vi "Configure Channel (OHM Scale).vi"(0 "VISA resource name":refnum<visa-resource-name>, 1 "Scaling":T2={"Floating point position (2)"=2, "Lower Scaling (0)"=0.0, "Upper Scaling (100.00)"=100.0, "Unit Character (\"\")"=""} {"Upper Scaling (100.00)" format="%_6g"; "Lower Scaling (0)" format="%_6g"; "Floating point position (2)" min=0 max=5 step=1}, 5 "Channel (0001)":string="0001", 7 "Enable Channel (True)":bool=TRUE, 9 "Type and Span":T1={"OHM Type (0 : 20ohm)"=0, "Enable Span (False)"=FALSE, "Lower Span (0.000)"=0.0, "Upper Span (20.000)"=20.0, "Bias (0)"=0.0} {"Bias (0)" format="%_6g"; "Upper Span (20.000)" min=-99999.0 max=99999.0 step=0.1 format="%.2f"; "Lower Span (0.000)" min=-99999.0 max=99999.0 step=0.1 format="%.2f"; "OHM Type (0 : 20ohm)" items=["20ohm", "200ohm", "2000ohm"]}, 11 "error in (no error)":errorcluster) -> (4 "VISA resource name out":refnum<visa-resource-name>, 6 "channel":string, 15 "error out":errorcluster)   [LabVIEW 2020, in "Yokogawa GX Series.lvlib"]
doc: "Sets the input range as OHM (for 4 wire RTD).\n\nCommand: SRangeAI"
uses:
  <instrlib>/Yokogawa GX Series/Yokogawa GX Series.lvlib
  <instrlib>/Yokogawa GX Series/Private/OHM Range.vi
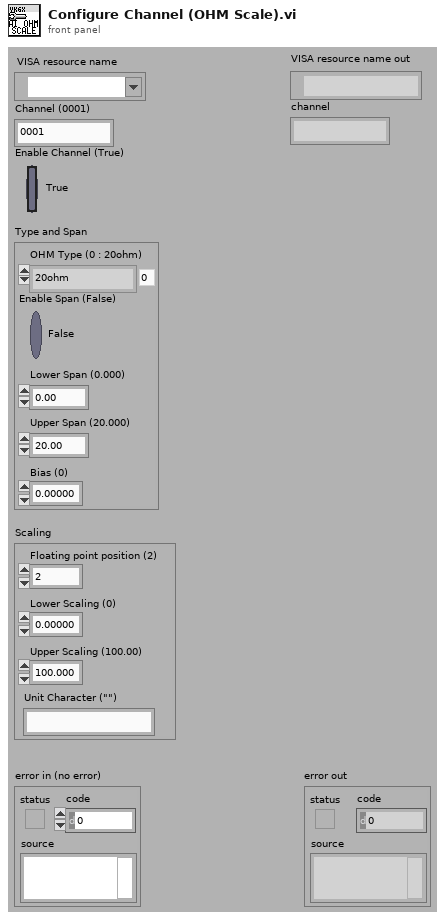
[diagram p1: front panel]
types:
  T1 = cluster{"OHM Type (0 : 20ohm)":i32, "Enable Span (False)":bool, "Lower Span (0.000)":dbl, "Upper Span (20.000)":dbl, "Bias (0)":dbl}
  T2 = cluster{"Floating point position (2)":i32, "Lower Scaling (0)":dbl, "Upper Scaling (100.00)":dbl, "Unit Character (\"\")":string}
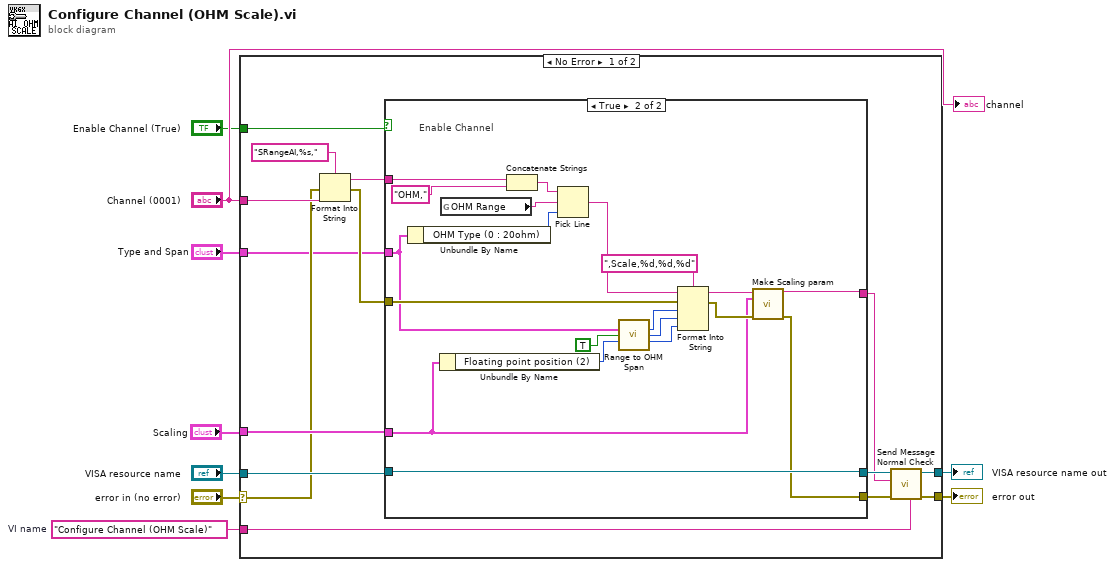
[diagram p0: block diagram]
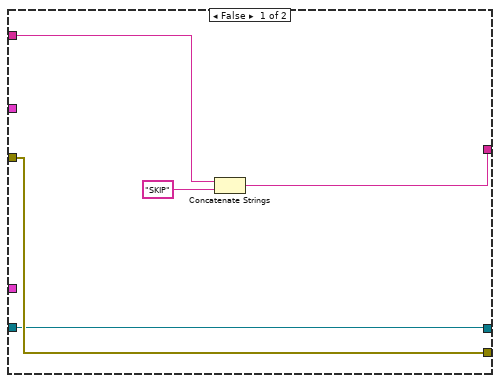
[diagram p2: hidden frame]
diagram:
  w3 = "Configure Channel (OHM Scale)"  # VI name
  n1 = case shown="No Error" "error in (no error)" {
    selector: "error in (no error)" -> [w11 w50]
    tunnel: "VISA resource name" -> [w21 w51]
    tunnel: [w18 w51] -> w8
    tunnel: [w17 w50] -> w7
    tunnel: "Scaling" -> [w15 _]
    tunnel: "Channel (0001)" -> [w14 _]
    tunnel: "Enable Channel (True)" -> [w13 _]
    tunnel: w3 -> [w12 _]
    tunnel: "Type and Span" -> [w10 _]
    frame No Error {
      n2 = Format Into String(format string="SRangeAI,%s,", error in=w11, w14) -> (resulting string=w22:string, error out=w23:errorcluster)  [unwired: 1 in]
      n3 = case shown="True" w13 {
        tunnel: w23 -> [w28 w41]
        tunnel: w22 -> [w29 w48]
        tunnel: [w28 w33] -> w19
        tunnel: w21 -> [w27 w42]
        tunnel: [w27 w42] -> w20
        tunnel: [w26 w34] -> w16
        tunnel: w15 -> [_ w35]
        tunnel: w10 -> [_ w30]
        frame False {
          n4 = Concatenate Strings(w29, "SKIP") -> (w26:string)
        }
        frame True {
          # "Enable Channel"
          n5 = Unbundle By Name(w30) -> ("OHM Type (0 : 20ohm)"=w46:i32)
          n6 = Unbundle By Name(w35) -> ("Floating point position (2)"=w39:i32)
          n7 = global read "OHM Range.vi" "OHM Range"() -> (w31:string)
          n8 = Concatenate Strings(w48, "OHM,") -> (w47:string)
          n9 = Pick Line(string ("")=w47, multi-line string=w31, line index=w46) -> (output string=w45:string)
          n10 = call <instrlib>:"Range to OHM Span.vi"("Range And Span"=w30, "Scaling? (False)"=TRUE, "Floating Point Position (2)"=w39) -> ("Lower Span"=w44:i32, "Upper Span"=w38:i32, "Bias"=w43:i32)  [unwired: 10 in]
          n11 = Format Into String(format string=",Scale,%d,%d,%d", initial string=w45, error in=w41, w44, w38, w43) -> (resulting string=w37:string, error out=w36:errorcluster)
          n12 = call <instrlib>:"Make Scaling param.vi"("String (\"\")"=w37, "Scaling"=w35, "error in (no error)"=w36) -> ("String After"=w34:string, "error out"=w33:errorcluster)  [unwired: 11 in]
        }
      }
      n13 = call <instrlib>:"Send Message Normal Check.vi"("Source (\"\")"=w12, "error in (no error)"=w19, "Send Message (\"\")"=w16, "VISA resource name"=w20) -> ("error out"=w17:errorcluster, "VISA resource name out"=w18:refnum<visa-resource-name>)  [unwired: 2 in, 4 out]
    }
    frame Error {
    }
  }
  "error out" <- w7
  "VISA resource name out" <- w8
  "channel" <- "Channel (0001)"
